vi "init.vi"(8 "error in":errorcluster, 10 "TBM module configuration in":refnum<class "TBM module configuration.lvclass">, 11 "OPC UA runtime in":refnum<class "OPC UA runtime.lvclass">) -> (0 "error out":errorcluster, 1 "data allocations":T1, 2 "execution settings":T4, 3 "OPC UA runtime out":refnum<class "OPC UA runtime.lvclass">)   [LabVIEW 2013, in "OPC UA runtime.lvclass"]
doc: "Provides an interface for initializing a module at runtime. While this interface performs no operations, a child should provide an override which may open any necessary references or sessions, allocate necessary memory, and perform any final configuration validataion before providing the full configuration <b>execution data</b> to the calling process."
uses:
  OPC UA runtime.lvclass
  <vilib>/NI/Tag Bus Module Framework/module configuration/TBM module configuration.lvclass
  <vilib>/NI/Tag Bus Module Framework/runtime/execution settings.ctl
  <vilib>/NI/Tag Bus Module Framework/channel/data tables.ctl
  <vilib>/NI/Tag Bus/dictionary/data dictionary.lvclass
  <vilib>/NI/Tag Bus/dictionary table pair.ctl
  <vilib>/NI/Tag Bus/table/data table.ctl
  configuration/OPC UA configuration.lvclass
  configuration/OPC UA configuration.lvclass/OPC UA configuration.ctl
  <vilib>/NI/Tag Bus Module Framework/channel/TBM channel.lvclass/TBM channel.ctl
  OPC UA runtime.lvclass/OPC UA runtime.ctl
  <vilib>/NI/Tag Bus/tag/Data Type.ctl
  configuration/OPC UA Data Type.ctl
  <vilib>/NI/Tag Bus/tag/tag descriptor.lvclass/tag descriptor.ctl
  <vilib>/NI/Tag Bus Module Framework/channel/TBM channel.lvclass
  <vilib>/NI/Tag Bus Module Framework/runtime/TBM module execution interface.lvclass
  <vilib>/NI/Tag Bus/tag/tag descriptor.lvclass
  <vilib>/NI/Tag Bus/tag bus.lvlib
  <vilib>/NI/Tag Bus/table/data table.lvlib
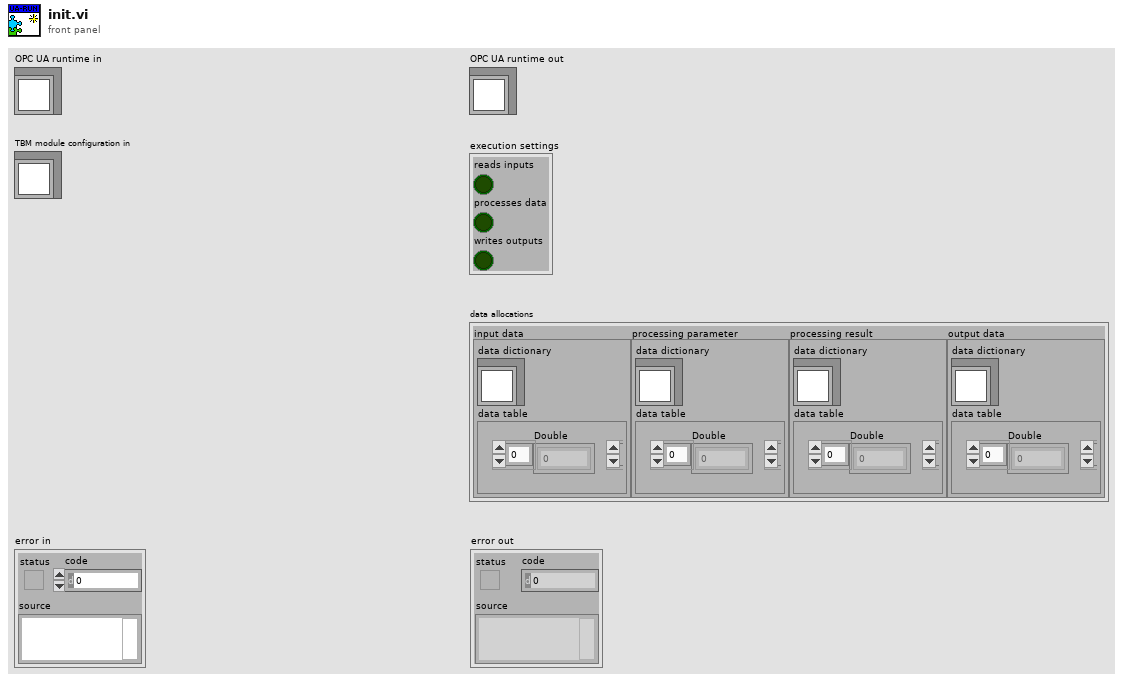
[diagram p1: front panel]
types:
  T1 = typedef "TBM channel.lvclass/data tables.ctl" = cluster{"input data":T2, "processing parameter":T2, "processing result":T2, "output data":T2}
  T2 = typedef "tag bus.lvlib/dictionary table pair.ctl" = cluster{"data dictionary":refnum<class "data dictionary.lvclass">, "data table":T3}
  T3 = typedef "tag bus.lvlib/data table.lvlib/data table.ctl" = cluster{"Double":dbl[], "Single":sgl[], "I64":i64[], "I32":i32[], "I16":i16[], "I8":i8[], "U64":u64[], "U32":u32[], "U16":u16[], "U8":u8[], "Boolean":bool[], "String":string[], "Array of Double":cluster{"DBL Array":dbl[]}[], "Array of Single":cluster{"SGL Array":sgl[]}[], "Array of I64":cluster{"I64 Array":i64[]}[], "Array of I32":cluster{"I32 Array":i32[]}[], "Array of I16":cluster{"I16 Array":i16[]}[], "Array of I8":cluster{"I8 Array":i8[]}[], "Array of U64":cluster{"U64 Array":u64[]}[], "Array of U32":cluster{"U32 Array":u32[]}[], "Array of U16":cluster{"U16 Array":u16[]}[], "Array of U8":cluster{"U8 Array":u8[]}[], "Array of Boolean":cluster{"Boolean Array":bool[]}[], "Array of String":cluster{"String Array":string[]}[]}
  T4 = typedef "TBM module execution interface.lvclass/execution settings.ctl" = cluster{"reads inputs":bool, "processes data":bool, "writes outputs":bool}
  T5 = typedef "tag bus.lvlib/tag descriptor.lvclass/Data Type.ctl" = enum16{"Double", "Single", "I64", "I32", "I16", "I8", "U64", "U32", "U16", "U8", "Boolean", "String", "Array of Double", "Array of Single", "Array of I64", "Array of I32", "Array of I16", "Array of I8", "Array of U64", "Array of U32", "Array of U16", "Array of U8", "Array of Boolean", "Array of String"}
  T6 = typedef "OPC UA configuration.lvclass/OPC UA Data Type.ctl" = u16
  T7 = cluster{"DCAF Data Type":T5, "Index":i32, "Node Path":string, "OPC UA Data Type":T6}
  T8 = typedef "OPC UA configuration.lvclass/Line.ctl" = cluster{"channel":refnum<class "TBM channel.lvclass">, "Node Path":string, "OPC UA Data Type":T6}
  T9 = typedef "TBM channel.lvclass/channel classification.ctl" = enum16{"input data", "output data", "processing parameter", "processing result"}
  T10 = cluster{"DCAF Data Type":T5, "Index":i32, "Node Path":string, "OPC UA Data Type":T6}[]
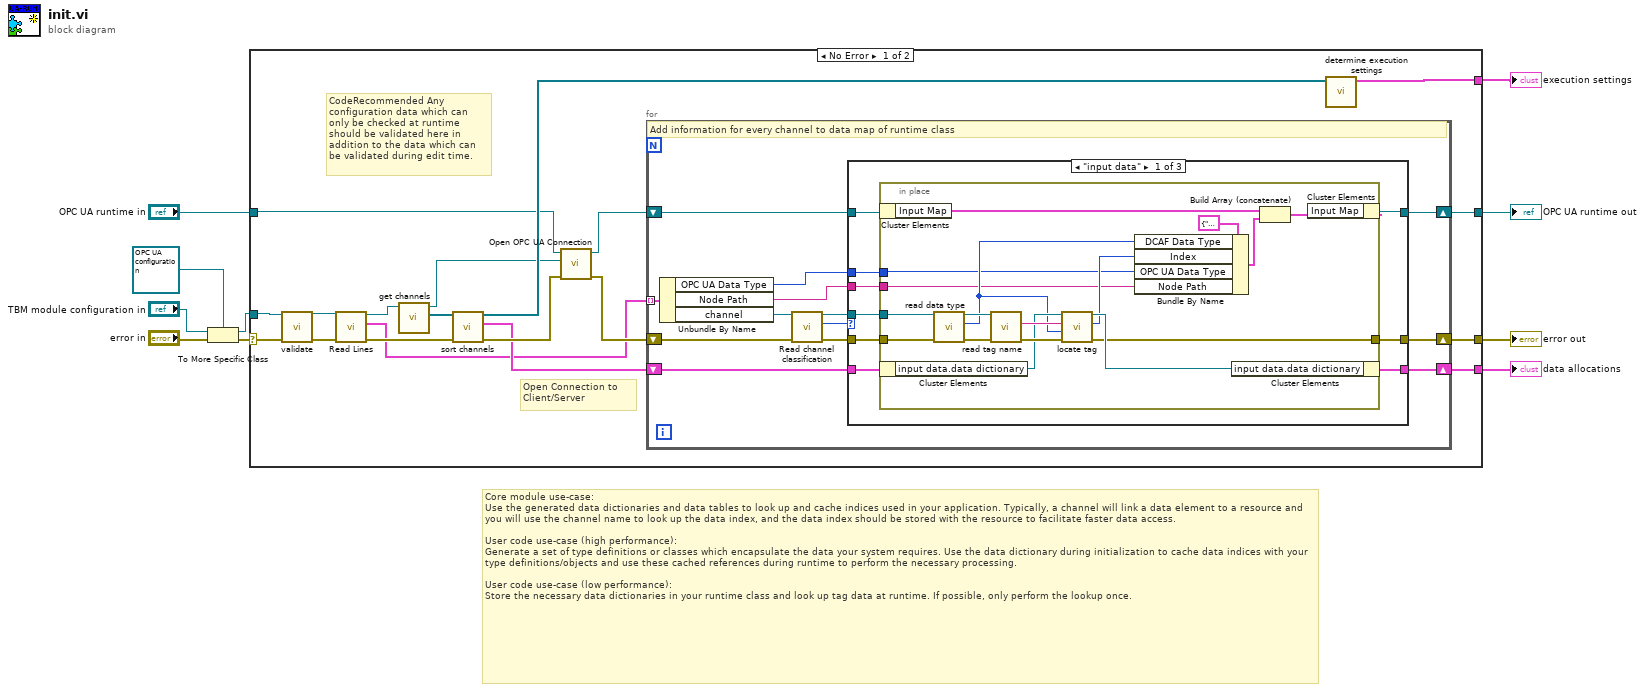
[diagram p0: block diagram]
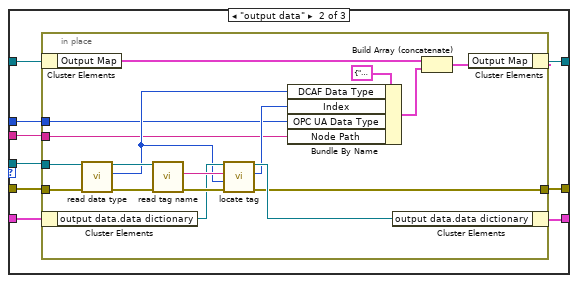
[diagram p2: hidden frame]
diagram:
  # "Core module use-case:\nUse the generated data dictionaries and data tables to look up and cache indices used in your application. Typically, a channel will link a data element to a resource and you will use the channel name to look up the data index, and the data index should be stored with the resource to facilitate faster data access.\n\nUser code use-case (high performance):\nGenerate a set of type definitions or classes which encapsulate the data your system requires. Use the data dictionary during initialization to cache data indices with your type definitions/objects and use these cached references during runtime to perform the necessary processing.\n\nUser code use-case (low performance):\nStore the necessary data dictionaries in your runtime class and look up tag data at runtime. If possible, only perform the lookup once."
  n1 = To More Specific Class(target class=refnum<class "OPC UA configuration.lvclass"> refnum ("Synchronous module configuration"), reference="TBM module configuration in", error in="error in") -> (specific class reference=w9:refnum<class "OPC UA configuration.lvclass">, error out=w10:errorcluster)
  n2 = case shown="No Error" w10 {
    selector: w10 -> [w28 w98]
    tunnel: w9 -> [w27 _]
    tunnel: "OPC UA runtime in" -> [w13 w99]
    tunnel: [w15 w99] -> w6
    tunnel: [w20 w98] -> w5
    tunnel: [w29 _] -> w4
    tunnel: [w14 _] -> w2
    frame No Error {
      # "CodeRecommended Any configuration data which can only be checked at runtime should be validated here in addition to the data which can be validated during edit time."
      # "Open Connection to\nClient/Server"
      n3 = call-dynamic "validate.vi"("error in"=w28, "OPC UA configuration in"=w27) -> ("error out"=w18:errorcluster, "OPC UA configuration out"=w12:refnum<class "OPC UA configuration.lvclass">)  [unwired: 8 in]
      n4 = call "Read Lines.vi"("error in (no error)"=w18, "OPC UA configuration in"=w12) -> ("error out"=w17:errorcluster, "Lines"=w16:T8[], "OPC UA configuration out"=w19:refnum<class "OPC UA configuration.lvclass">)  [unwired: 7 in]
      n5 = call-dynamic "get channels.vi"("OPC UA configuration in"=w19) -> ("channels"=w26:refnum<class "TBM channel.lvclass">[], "OPC UA configuration out"=w11:refnum<class "OPC UA configuration.lvclass">)  [unwired: 9 in]
      n6 = call <vilib>:"sort channels.vi"("error in"=w17, "channels in"=w26) -> ("error out"=w25:errorcluster, "data allocations"=w21:T1, "channels out"=w22:refnum<class "TBM channel.lvclass">[])  [unwired: 7 in]
      n7 = call "Open OPC UA Connection.vi"("error in (no error)"=w25, "OPC UA configuration"=w11, "OPC UA runtime in"=w13) -> ("error out"=w24:errorcluster, "OPC UA runtime out"=w23:refnum<class "OPC UA runtime.lvclass">)  [unwired: 7 in]
      n8 = for {
        shift-right: [w36] -> w20
        shift-left: w24 -> [w42]
        shift-right: [w38] -> w15
        shift-left: w23 -> [w37]
        shift-right: [w34] -> w14
        shift-left: w21 -> [w35]
        tunnel: w16 -> [w33] mode=indexing
        # "Add information for every channel to data map of runtime class"
        n9 = Unbundle By Name(w33) -> ("OPC UA Data Type"=w30:T6, "Node Path"=w31:string, "channel"=w32:refnum<class "TBM channel.lvclass">)
        n10 = call <vilib>:"Read channel classification.vi"("error in"=w42, "channel in"=w32) -> ("error out"=w39:errorcluster, "channel classification"=w41:T9, "channel out"=w40:refnum<class "TBM channel.lvclass">)  [unwired: 7 in]
        n11 = case shown="\"input data\"" w41 {
          tunnel: w40 -> [w48 w75 _]
          tunnel: w39 -> [w49 w74 w96]
          tunnel: [w45 w70 w97] -> w38
          tunnel: w37 -> [w51 w77 w97]
          tunnel: [w47 w71 w96] -> w36
          tunnel: w35 -> [w50 w73 w95]
          tunnel: [w46 w72 w95] -> w34
          tunnel: w31 -> [w44 w76 _]
          tunnel: w30 -> [w43 w69 _]
          frame "input data" {
            n12 = in-place {
              in-place-border: w49 -> [w64]
              in-place-border: w48 -> [w66]
              in-place-border: [w56] -> w47
              in-place-border: w44 -> [w55]
              in-place-border: w43 -> [w52]
              n13 = in-place-cluster #1(w51) -> ("Input Map"=w67:T10)
              n14 = in-place-cluster #2(w50) -> ("input data.data dictionary"=w60:refnum<class "data dictionary.lvclass">)
              n15 = call <vilib>:"read data type.vi"("error in"=w64, "system tag in"=w66) -> ("error out"=w65:errorcluster, "data type"=w59:T5, "system tag out"=w61:refnum<class "TBM channel.lvclass">)  [unwired: 7 in]
              n16 = call <vilib>:"read tag name.vi"("error in"=w65, "system tag in"=w61) -> ("error out"=w63:errorcluster, "name"=w62:string)  [unwired: 7 in, 1 out]
              n17 = call <vilib>:"locate tag.vi"("error in"=w63, "data type"=w59, "name"=w62, "data dictionary in"=w60) -> ("error out"=w56:errorcluster, "index"=w57:i32, "data dictionary out"=w58:refnum<class "data dictionary.lvclass">)  [unwired: 5 in]
              n18 = Bundle By Name(cluster=T7 {"DCAF Data Type"=enum."Double", "Index"=0, "Node Path"="", "OPC UA Data Type"=0} ("Item"), "DCAF Data Type"=w59, "Index"=w57, "OPC UA Data Type"=w52, "Node Path"=w55) -> (w54:T7)
              n19 = in-place-cluster #2("input data.data dictionary"=w58) -> (w46:T1)
              n20 = Build Array (concatenate)(w67, w54) -> (w68:T10)
              n21 = in-place-cluster #1("Input Map"=w68) -> (w45:refnum<class "OPC UA runtime.lvclass">)
            }
          }
          frame "output data" {
            n22 = in-place {
              in-place-border: w74 -> [w90]
              in-place-border: w75 -> [w92]
              in-place-border: [w82] -> w71
              in-place-border: w76 -> [w80]
              in-place-border: w69 -> [w79]
              n23 = in-place-cluster #3(w77) -> ("Output Map"=w93:T10)
              n24 = in-place-cluster #4(w73) -> ("output data.data dictionary"=w86:refnum<class "data dictionary.lvclass">)
              n25 = call <vilib>:"read data type.vi"("error in"=w90, "system tag in"=w92) -> ("error out"=w91:errorcluster, "data type"=w85:T5, "system tag out"=w87:refnum<class "TBM channel.lvclass">)  [unwired: 7 in]
              n26 = call <vilib>:"read tag name.vi"("error in"=w91, "system tag in"=w87) -> ("error out"=w89:errorcluster, "name"=w88:string)  [unwired: 7 in, 1 out]
              n27 = call <vilib>:"locate tag.vi"("error in"=w89, "data type"=w85, "name"=w88, "data dictionary in"=w86) -> ("error out"=w82:errorcluster, "index"=w83:i32, "data dictionary out"=w84:refnum<class "data dictionary.lvclass">)  [unwired: 5 in]
              n28 = Bundle By Name(cluster=T7 {"DCAF Data Type"=enum."Double", "Index"=0, "Node Path"="", "OPC UA Data Type"=0} ("Item"), "DCAF Data Type"=w85, "Index"=w83, "OPC UA Data Type"=w79, "Node Path"=w80) -> (w81:T7)
              n29 = in-place-cluster #4("output data.data dictionary"=w84) -> (w72:T1)
              n30 = Build Array (concatenate)(w93, w81) -> (w94:T10)
              n31 = in-place-cluster #3("Output Map"=w94) -> (w70:refnum<class "OPC UA runtime.lvclass">)
            }
          }
          frame Default {
          }
        }
      }
      n32 = call <vilib>:"determine execution settings.vi"("channels"=w22) -> ("execution settings"=w29:T4)  [unwired: 10 in]
    }
    frame Error {
    }
  }
  "error out" <- w5
  "OPC UA runtime out" <- w6
  "execution settings" <- w4
  "data allocations" <- w2
